vi "configure.vi"(8 "error in (no error)":errorcluster, 9 "Value":i32, 10 "ILC":refnum<class "ILC.lvclass">, 11 "ConfigureILCCH0 in":refnum<class "ConfigureILCCH0Strategy.lvclass">) -> (0 "error out":errorcluster, 3 "ConfigureILCCH0 out":refnum<class "ConfigureILCCH0Strategy.lvclass">)   [LabVIEW 2015, in "ConfigureILCCH0Strategy.lvclass"]
uses:
  ConfigureILCCH0Strategy.lvclass
  <userlib>/Common/ILC/ILC/ILC.lvclass
  <userlib>/Common/ILC/ILC/ILC.lvclass/ILC.ctl
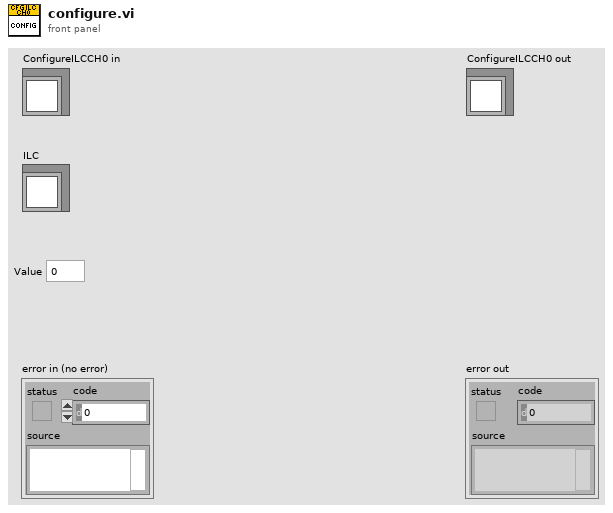
[diagram p1: front panel]
types:
  T1 = typedef "ILCCommon.lvlib/ILCTypedefs.lvlib/OutputData.ctl" = cluster{"Step & Direction":i16, "Blower RPM":u8, "PWM (SSR)":u8, "Ch1":u16, "Ch2":u16, "Ch3":u16, "Ch4":u16}
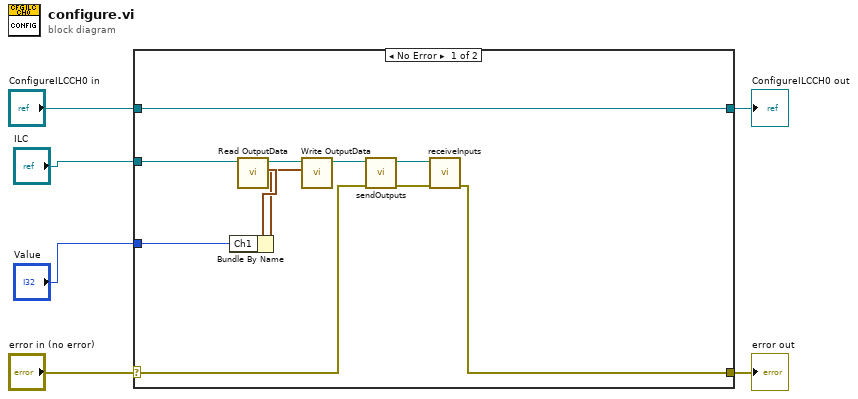
[diagram p0: block diagram]
diagram:
  n1 = case shown="No Error" "error in (no error)" {
    selector: "error in (no error)" -> [w9 w19]
    tunnel: [w7 w19] -> w5
    tunnel: [w17 w18] -> w3
    tunnel: "ConfigureILCCH0 in" -> [w17 w18]
    tunnel: "ILC" -> [w16 _]
    tunnel: "Value" -> [w14 _]
    frame No Error {
      n2 = call <userlib>:"Read OutputData.vi"("ILC in"=w16) -> ("OutputData"=w15:T1, "ILC out"=w12:refnum<class "ILC.lvclass">)  [unwired: 9 in]
      n3 = Bundle By Name(cluster=w15, "Ch1"=w14) -> (w13:T1)
      n4 = call <userlib>:"Write OutputData.vi"("OutputData"=w13, "ILC in"=w12) -> ("ILC out"=w11:refnum<class "ILC.lvclass">)  [unwired: 9 in]
      n5 = call <userlib>:"sendOutputs.vi"("error in (no error)"=w9, "ILC in"=w11) -> ("error out"=w8:errorcluster, "ILC out"=w10:refnum<class "ILC.lvclass">)  [unwired: 8 in]
      n6 = call <userlib>:"receiveInputs.vi"("error in (no error)"=w8, "ILC in"=w10) -> ("error out"=w7:errorcluster)  [unwired: 6 in, 3 out]
    }
    frame Error {
    }
  }
  "error out" <- w5
  "ConfigureILCCH0 out" <- w3
